vi "Alignment.vi"(0 "Range":dbl=30.0 format="%#_13g", 1 "Target":dbl format="%#_13g", 2 "Camera Feedback":dbl=57.947591168268985 format="%#_13g", 3 "RightMotorSpeed":dbl format="%#_13g", 4 "LeftMotorSpeed":dbl format="%#_13g", 5 "POV":i32=180, 9 "Turn_Gain":dbl=0.2 format="%#_13g") -> (15 "Right Motor":dbl=-0.25 format="%#_13g", 17 "LeftAndRight?":bool, 18 "Left Motor":dbl=0.25 format="%#_13g")   [LabVIEW 2016]
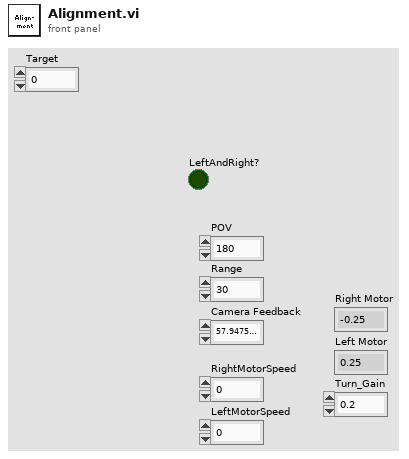
[diagram p1: front panel]
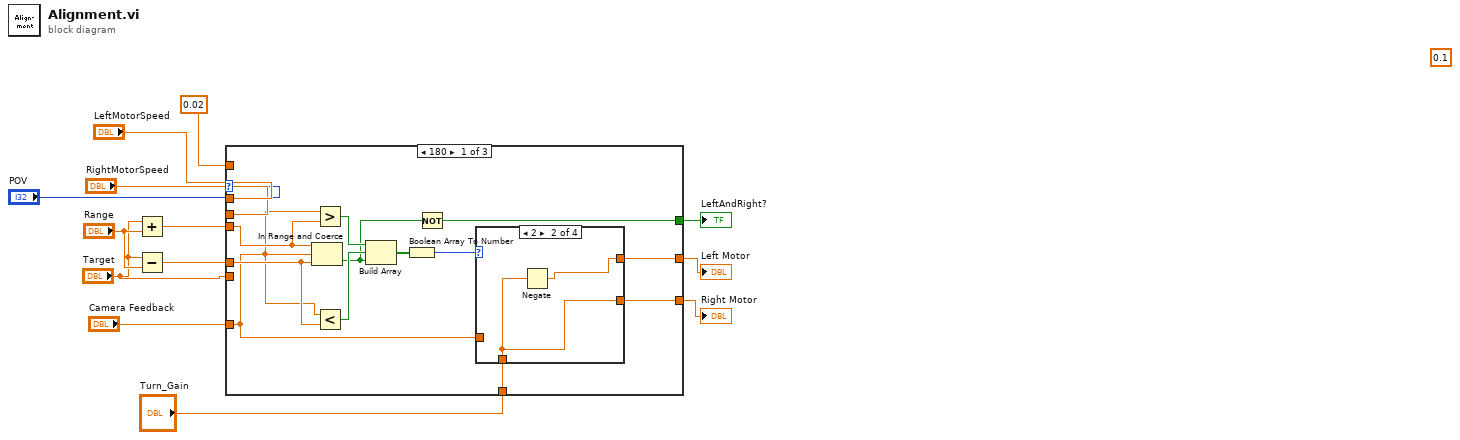
[diagram p0: block diagram]
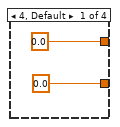
[diagram p2: hidden frame]
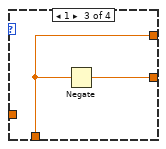
[diagram p3: hidden frame]
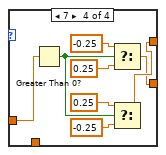
[diagram p4: hidden frame]
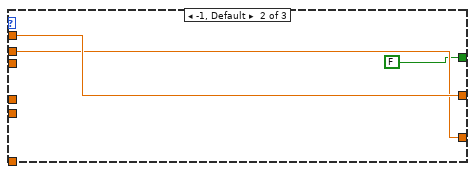
[diagram p5: hidden frame]
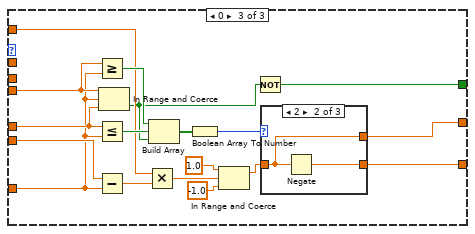
[diagram p6: hidden frame]
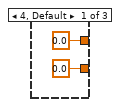
[diagram p7: hidden frame]
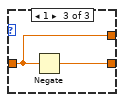
[diagram p8: hidden frame]
diagram:
  (unwired) 0.1 ("Range")
  n1 = Add(x="Target", y="Range") -> (x+y=w7:dbl)
  n2 = Subtract(x="Target", y="Range") -> (x-y=w6:dbl)
  n3 = case shown="180" "POV" {
    tunnel: [w22 w42 w56] -> w13
    tunnel: "LeftMotorSpeed" -> [_ w42 _]
    tunnel: [w23 w41 w57] -> w11
    tunnel: "RightMotorSpeed" -> [_ w41 _]
    tunnel: "Camera Feedback" -> [w16 _ w51]
    tunnel: w7 -> [w18 _ w55]
    tunnel: w6 -> [w17 _ w60]
    tunnel: [w15 FALSE w43] -> w4
    tunnel: "Target" -> [_ _ w52]
    tunnel: 0.02 -> [_ _ w49]
    tunnel: "Turn_Gain" -> [w14 _ _]
    frame 180 {
      n4 = In Range and Coerce(upper limit=w18, x=w16, lower limit=w17) -> (In Range?=w19:bool)  [unwired: 1 out]
      n5 = Greater?(x=w16, y=w18) -> (0:w21:bool)
      n6 = Less?(x=w16, y=w17) -> (x < y?=w20:bool)
      n7 = Build Array(w21, w20, w19) -> (w25:bool[])
      n8 = Boolean Array To Number(Boolean array=w25) -> (number=w24:u32)
      n9 = Not(x=w19) -> (.not. x?=w15:bool)
      n10 = case shown="2" w24 {
        tunnel: [0.0 w29 w31 w37] -> w23
        tunnel: [0.0 w28 w30 w38] -> w22
        tunnel: w16 -> [_ _ _ w32]
        tunnel: w14 -> [_ w29 w30 _]
        frame 4, Default {
        }
        frame 2 {
          n11 = Negate(x=w29) -> (-x=w28:dbl)
        }
        frame 1 {
          n12 = Negate(x=w30) -> (-x=w31:dbl)
        }
        frame 7 {
          n13 = Greater Than 0?(x=w32) -> (x > 0?=w39:bool)
          n14 = Select(t=-0.25, s=w39, f=0.25 ("t")) -> (s? t:f=w37:dbl)
          n15 = Select(t=0.25, s=w39, f=-0.25 ("t")) -> (s? t:f=w38:dbl)
        }
      }
    }
    frame -1, Default {
    }
    frame 0 {
      n16 = Greater Or Equal?(x=w55, y=w51) -> (x >= y?=w54:bool)
      n17 = Less Or Equal?(x=w60, y=w51) -> (x <= y?=w53:bool)
      n18 = Subtract(x=w52, y=w51) -> (x-y=w50:dbl)
      n19 = In Range and Coerce(upper limit=w55, x=w51, lower limit=w60) -> (In Range?=w44:bool)  [unwired: 1 out]
      n20 = Multiply(x=w49, y=w50) -> (x*y=w48:dbl)
      n21 = Build Array(w54, w53, w44) -> (w59:bool[])
      n22 = Boolean Array To Number(Boolean array=w59) -> (number=w58:u32)
      n23 = In Range and Coerce(upper limit=1.0, x=w48, lower limit=-1.0) -> (coerced(x)=w47:dbl)  [unwired: 1 out]
      n24 = Not(x=w44) -> (.not. x?=w43:bool)
      n25 = case shown="2" w58 {
        tunnel: [0.0 w63 w65] -> w57
        tunnel: [0.0 w64 w66] -> w56
        tunnel: w47 -> [_ w64 w66]
        frame 4, Default {
        }
        frame 2 {
          n26 = Negate(x=w64) -> (-x=w63:dbl)
        }
        frame 1 {
          n27 = Negate(x=w66) -> (-x=w65:dbl)
        }
      }
    }
  }
  "Left Motor" <- w13
  "Right Motor" <- w11
  "LeftAndRight?" <- w4
